vi "Read.vi"() -> ()   [LabVIEW 2018]
uses:
  Class/Seimens.lvclass
  Class/Public/Read/SeimensS7Net_ReadInt16[].vi
  Class/Public/Write/SeimensS7Net_WriteBool.vi
panel:
  in  "value":bool
  in  "Write":bool
  in  "Read":bool
  in  "停止":bool
  in  "WriteAddress":string="DB600.0"
  in  "error in (no error)":errorcluster caption="错误输入（无错误）"
  out "error out":errorcluster caption="错误输出"
  in  "ReadAddress":string="DB600.0"
  in  "ReadLength":u16=1000
  out "ReadArray":i16[](array[numeric])
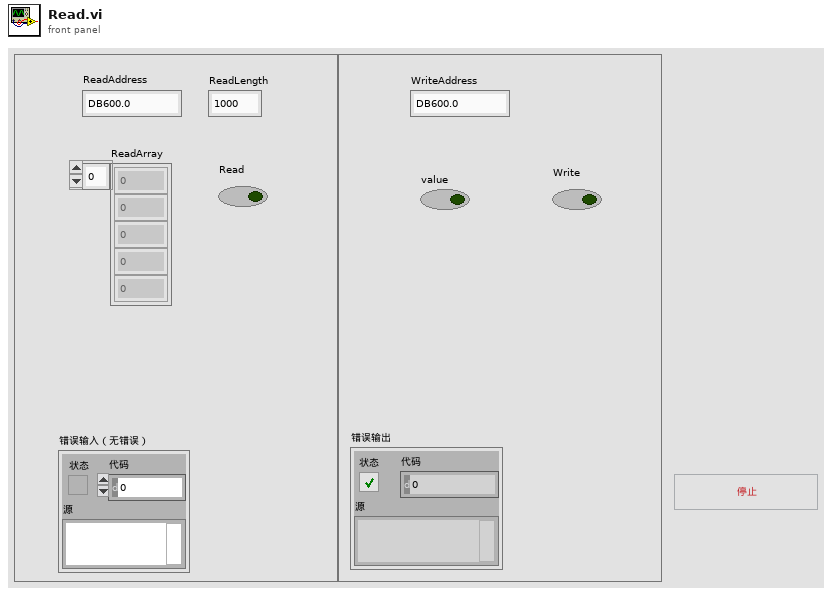
[diagram p1: front panel]
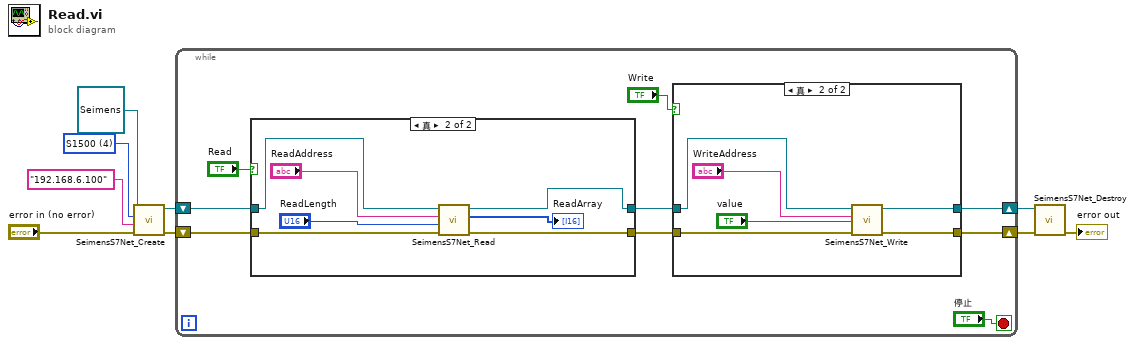
[diagram p0: block diagram]
diagram:
  w6 = 4 items=["S1200"=1, "S300"=2, "S400"=3, "S1500"=4, "S200Smart"=5, "S200"=6] ("siemens")
  n1 = call "SeimensS7Net_Create.vi"("error in (no error)"="error in (no error)", "ipAddress"="192.168.6.100", "siemens"=w6, "Seimens 输入"=refnum<class "Seimens.lvclass"> refnum) -> ("error out"=w9:errorcluster, "Seimens 输出"=w8:refnum<class "Seimens.lvclass">)  [unwired: 6 in]
  n2 = while {
    shift-right: [w15] -> w3
    shift-left: w9 -> [w18]
    shift-right: [w13] -> w2
    shift-left: w8 -> [w17]
    stop <- "停止" stop-if-true
    n3 = case shown="真" "Read" {
      tunnel: w18 -> [w19 w27]
      tunnel: w17 -> [w20 w26]
      tunnel: [w19 w22] -> w16
      tunnel: [w20 w21] -> w14
      frame False {
      }
      frame True {
        n4 = call-poly "SeimensS7Net_Read.vi"("error in (no error)"=w27, "length"="ReadLength", "address"="ReadAddress", "Seimens 输入"=w26) -> ("error out"=w22:errorcluster, "ReadArray"=→"ReadArray":i16[], "Seimens 输出"=w21:refnum<class "Seimens.lvclass">)  [unwired: 5 in]
      }
    }
    n5 = case shown="真" "Write" {
      tunnel: w16 -> [w28 w35]
      tunnel: [w28 w34] -> w15
      tunnel: w14 -> [w29 w33]
      tunnel: [w29 w32] -> w13
      frame False {
      }
      frame True {
        n6 = call-poly "SeimensS7Net_Write.vi"("error in (no error)"=w35, "value"="value", "address"="WriteAddress", "Seimens 输入"=w33) -> ("error out"=w34:errorcluster, "Seimens 输出"=w32:refnum<class "Seimens.lvclass">)  [unwired: 6 in]
      }
    }
  }
  n7 = call "SeimensS7Net_Destroy.vi"("error in (no error)"=w3, "Seimens 输入"=w2) -> ("error out"=→"error out":errorcluster)  [unwired: 9 in]
